vi "IntensityGraphOp_Dialog.vi"(1 "stop":bool, 2 "Op-Mode":T1(ring)) -> (0 "Op-Mode output":T1(ring))   [LabVIEW 2020]
panel:
  # "Choose an Operator:"
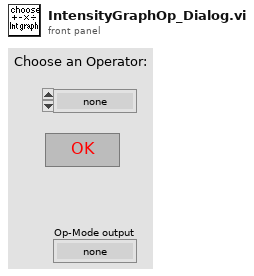
[diagram p1: front panel]
types:
  T1 = enum16{"none", " + ", " - ", " * ", " / ", "Integral", "Differential", "FFT"}
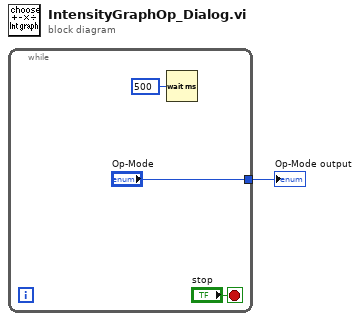
[diagram p0: block diagram]
diagram:
  n1 = while {
    tunnel: ["Op-Mode"] -> w1
    stop <- "stop" stop-if-true
    n2 = Wait (ms)(milliseconds to wait=u32 500) -> ()  [unwired: 1 out]
  }
  "Op-Mode output" <- w1
